vi "Check Queue Space.vi"(9 "Timeout mS":i32, 11 "Queues In":refnum<queue>[](array[refnum])) -> (1 "Timeout":bool, 3 "Queues":refnum<queue>[](array[refnum]))   [LabVIEW 2020, in "Connection.lvclass"]
uses:
  Connection.lvclass
  Connection.lvclass/Connection.ctl
  Element.ctl
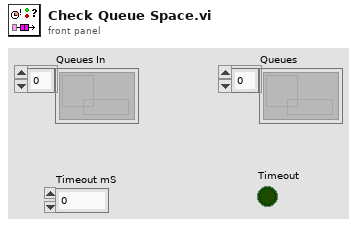
[diagram p1: front panel]
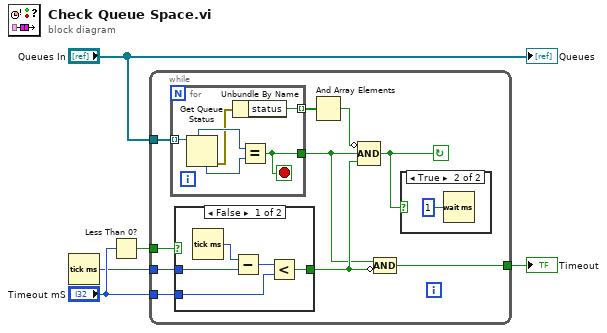
[diagram p0: block diagram]
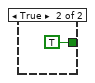
[diagram p2: hidden frame]
diagram:
  n1 = Tick Count (ms)() -> (millisecond timer value=w2:u32)
  n2 = Less Than 0?(x="Timeout mS") -> (x < 0?=w4:bool)
  n3 = while {
    tunnel: "Queues In" -> [w15]
    tunnel: w2 -> [w14]
    tunnel: "Timeout mS" -> [w13]
    tunnel: [w7] -> w1
    tunnel: w4 -> [w9]
    stop <- w12 continue-if-true
    n4 = for {
      tunnel: w15 -> [w27] mode=indexing
      tunnel: [w24] -> w6
      tunnel: [w22] -> w11 mode=indexing
      stop <- w24 stop-if-true
      n5 = Get Queue Status(queue=w27) -> (max queue size=w26:i32, error out=w23:errorcluster, # elements in queue=w25:i32)  [unwired: 2 in, 5 out]
      n6 = Unbundle By Name(w23) -> ("status"=w22:bool)
      n7 = Equal?(x=w26, y=w25) -> (x = y?=w24:bool)
    }
    n8 = case shown="False" w9 {
      tunnel: w14 -> [w20 _]
      tunnel: w13 -> [w17 _]
      tunnel: [w16 TRUE] -> w8
      frame False {
        n9 = Tick Count (ms)() -> (millisecond timer value=w19:u32)
        n10 = Subtract(x=w19, y=w20) -> (x-y=w18:u32)
        n11 = Less?(x=w18, y=w17) -> (x < y?=w16:bool)
      }
      frame True {
      }
    }
    n12 = And Array Elements(Boolean array=w11) -> (logical AND=w10:bool)
    n13 = Compound Arithmetic op=AND(invert w10, w6, w8) -> (w12:bool)
    n14 = Compound Arithmetic op=AND(w6, invert w8) -> (w7:bool)
    n15 = case shown="True" w12 {
      frame False {
      }
      frame True {
        n16 = Wait (ms)(milliseconds to wait=u32 1) -> ()  [unwired: 1 out]
      }
    }
  }
  "Timeout" <- w1
  "Queues" <- "Queues In"
